vi "tra25cc_wait_for_state.vi"(8 "error in (no error)":errorcluster, 9 "xyz/xy":bool=TRUE, 10 "state_to_wait":u32(ring)=50 items=["READY from HOMING"=50], 11 "conn_xyz_in":T2) -> (0 "error out":errorcluster, 2 "state_xyz":cluster{u32, u32, u32}, 3 "conn_xyz_out":T1)   [LabVIEW 2018]
uses:
  D:/Data/Thea/tests/Labview/Scanner_v3_Phy-2019.05.06/src/Stage_xyz/Dll/Newport.CONEXCC.CommandInterface.dll
  Dll/Newport.CONEXCC.CommandInterface.dll
  <vilib>/Platform/TimedLoop/XDataNode/timing_clust.ctl
  <vilib>/Platform/TimedLoop/XDataNode/nitl_modes.ctl
  <vilib>/Platform/TimedLoop/XDataNode/wakeup.ctl
  <vilib>/platform/TimedLoop/XDataNode/XDataNode.xnode
  <vilib>/Platform/TimedLoop/XDataNode/XDNodeRunTimeDep.lvlib
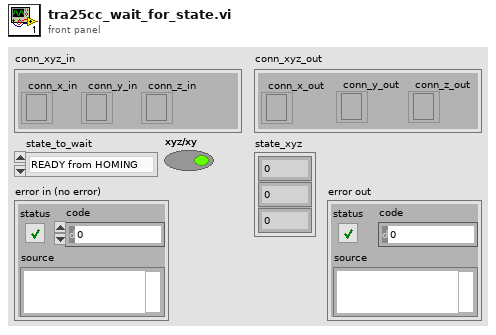
[diagram p1: front panel]
types:
  T1 = cluster{"conn_x_out":refnum<k24>, "conn_y_out":refnum<k24>, "conn_z_out":refnum<k24>}
  T2 = cluster{"conn_x_in":refnum<k24>, "conn_y_in":refnum<k24>, "conn_z_in":refnum<k24>}
  T3 = typedef "XDNodeRunTimeDep.lvlib/timing_clust.ctl" = cluster{"Expected End [f-1]":u64, "Actual End [f-1]":u64, "Finished Late? [f-1]":bool, "Expected End [i-1]":u64, "Actual End [i-1]":u64, "Finished Late? [i-1]":bool, "Expected Start [i]":u64, "Actual Start [i]":u64, "Expected Start [f]":u64, "Actual Start [f]":u64, "Source Name":string, "Structure Name":string, "Period":i64, "Deadline":i64, "Offset":i64, "Start":i64, "Priority":i32, "Timeout":i32, "Mode":T4, "Wakeup Reason":T5, "Error":errorcluster, "Source Type":string, "Secondary Source Type":string, "Global End Time":u64, "Global Start Time":u64, "Frame Duration":u64, "Iteration Duration":u64, "Assigned CPU":i32, "I/O Scan Engine Mode":u32}
  T4 = typedef "XDNodeRunTimeDep.lvlib/nitl_modes.ctl" = enum32{"No Change", "Process missed periods, maintain original phase", "Discard missed periods, maintain original phase", "Process missed periods, ignore original phase", "Discard missed periods, ignore original phase"}
  T5 = typedef "XDNodeRunTimeDep.lvlib/wakeup.ctl" = enum32{"Normal", "Aborted", "Asynchronous wakeup", "Timing source error", "Timed loop error", "Timeout"}
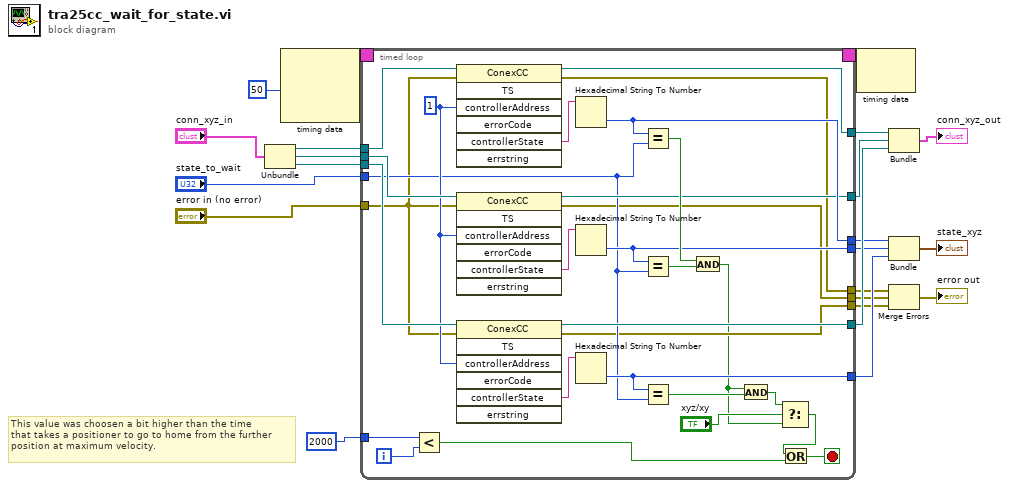
[diagram p0: block diagram]
diagram:
  # "This value was choosen a bit higher than the time\nthat takes a positioner to go to home from the further\nposition at maximum velocity."
  n1 = Unbundle("conn_xyz_in") -> ("conn_x_in"=w18:refnum<k24>, "conn_y_in"=w16:refnum<k24>, "conn_z_in"=w15:refnum<k24>)
  n2 = node-c288(i64 50 ("Period")) -> (w22:T3)  [unwired: 2 in]
  n3 = timed-loop {
    timing: w22 -> [_]
    timing-out: [_] -> w21
    tunnel: [w51] -> w17
    tunnel: w18 -> [w50]
    tunnel: [w48] -> w12
    tunnel: "state_to_wait" -> [w34]
    tunnel: w16 -> [w46]
    tunnel: w15 -> [w45]
    tunnel: [w38] -> w11
    tunnel: [w37] -> w10
    tunnel: [w36] -> w14
    tunnel: [w35] -> w13
    tunnel: [w33] -> w7
    tunnel: [w32] -> w9
    tunnel: [w31] -> w8
    tunnel: "error in (no error)" -> [w30]
    tunnel: 2000 ("x") -> [w27]
    i -> [w29]
    stop <- w47 stop-if-true
    w39 = 1 ("controllerAddress")
    n4 = Less?(x=w27, y=w29) -> (x < y?=w28:bool)
    n5 = invoke class="ConexCC" method="TS"(reference=w50, error in=w30, "controllerAddress"=w39) -> (reference out=w51:refnum<k24>, error out=w33:errorcluster, "controllerState"=w49:string)  [unwired: 4 in, 4 out]
    n6 = invoke class="ConexCC" method="TS"(reference=w46, error in=w30, "controllerAddress"=w39) -> (reference out=w36:refnum<k24>, error out=w32:errorcluster, "controllerState"=w44:string)  [unwired: 4 in, 4 out]
    n7 = invoke class="ConexCC" method="TS"(reference=w45, error in=w30, "controllerAddress"=w39) -> (reference out=w35:refnum<k24>, error out=w31:errorcluster, "controllerState"=w43:string)  [unwired: 4 in, 4 out]
    n8 = Hexadecimal String To Number(string=w49) -> (number=w48:u32)  [unwired: 2 in, 1 out]
    n9 = Hexadecimal String To Number(string=w44) -> (number=w38:u32)  [unwired: 2 in, 1 out]
    n10 = Hexadecimal String To Number(string=w43) -> (number=w37:u32)  [unwired: 2 in, 1 out]
    n11 = Equal?(x=w48, y=w34) -> (x = y?=w41:bool)
    n12 = Equal?(x=w38, y=w34) -> (x = y?=w42:bool)
    n13 = Equal?(x=w37, y=w34) -> (x = y?=w40:bool)
    n14 = And(x=w41, y=w42) -> (x .and. y?=w23:bool)
    n15 = And(x=w23, y=w40) -> (x .and. y?=w24:bool)
    n16 = Select(t=w24, s="xyz/xy", f=w23) -> (s? t:f=w25:bool)
    n17 = Or(x=w25, y=w28) -> (x .or. y?=w47:bool)
  }
  n18 = node-c288(w21) -> ()  [unwired: 1 out]
  n19 = Bundle("conn_x_in"=w17, "conn_y_in"=w14, "conn_z_in"=w13) -> (→"conn_xyz_out":T2)  [unwired: 1 in]
  n20 = Bundle(w12, w11, w10) -> (→"state_xyz":cluster{u32, u32, u32})  [unwired: 1 in]
  n21 = Merge Errors(w7, w9, w8) -> (→"error out":errorcluster)
